vi "Get Type Specializations.vi"(8 "error in":errorcluster, 11 "Continuous Counting Mesurement2 in":refnum<class "Continuous Counting Measurement2.lvclass">) -> (0 "error out":errorcluster, 2 "type specializations":T1[](array[typedef]), 3 "Continuous Counting Mesurement2 out":refnum<class "Continuous Counting Measurement2.lvclass">)   [LabVIEW 2021, in "MeasurementServerTests.lvlib" / "Measurement Service Tests.lvlib" / "Continuous Counting Measurement2.lvclass"]
doc: "Provides optional metadata used to describe type specializations for measurement inputs and outputs that can be utilized by the user interface. For example, by specifying an input as an ioresource for a particular type of instrument, the user interface can limit selection of I/O resources to those that belong to that instrument type."
uses:
  Continuous Counting Measurement2.lvclass
  Runtime/Measurements/Helpers/TypeDefs/Parameter Type Specialization.ctl
  Runtime/Measurements/Helpers/TypeDefs/Type Specialization.ctl
  Runtime/Measurements/Helpers/TypeDefs/Type Specialization Key.ctl
  Runtime/Measurements/NI Measurement Plug-In SDK.lvlib
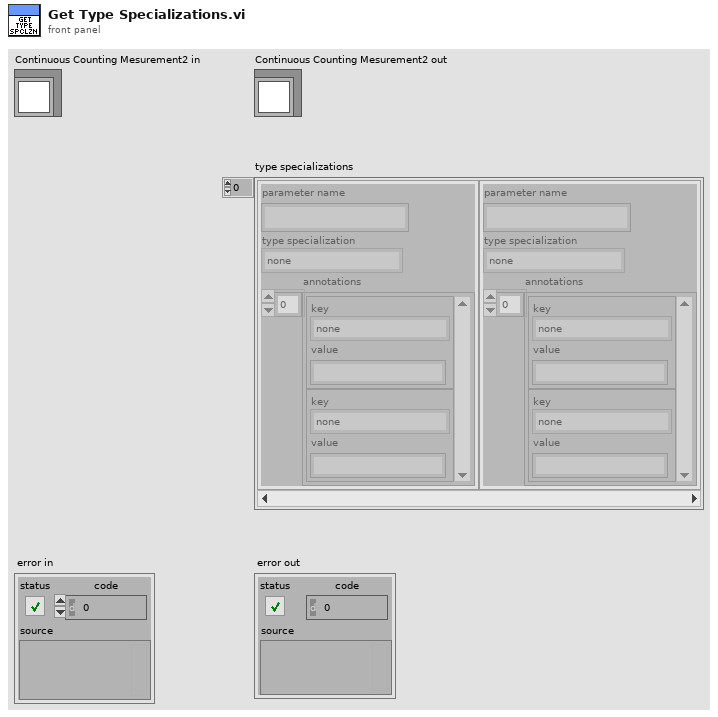
[diagram p1: front panel]
types:
  T1 = typedef "NI Measurement Plug-In SDK.lvlib/Parameter Type Specialization.ctl" = cluster{"parameter name":string, "type specialization":T2, "annotations":cluster{"key":T3, "value":string}[]}
  T2 = typedef "NI Measurement Plug-In SDK.lvlib/Type Specialization.ctl" = enum16{"none", "pin", "path", "enum", "ioresource"}
  T3 = typedef "NI Measurement Plug-In SDK.lvlib/Type Specialization Key.ctl" = enum16{"none", "pin.instrument_type", "enum.values", "ioresource.instrument_type"}
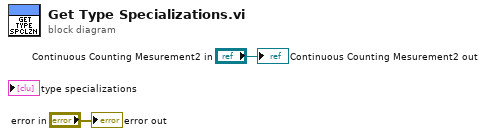
[diagram p0: block diagram]
diagram:
  "error out" <- "error in"
  "Continuous Counting Mesurement2 out" <- "Continuous Counting Mesurement2 in"
